vi "Serial Numbers.vi"(11 "Total Number of Units":i32=1 min=1 max=32 step=1) -> (2 "Serial Numbers":string[](array[string]))   [LabVIEW 2024]
panel:
  in  "Serial Number":string
  in  "Enter":bool
  out "Current Unit":i32
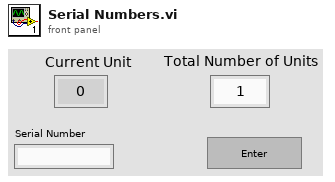
[diagram p1: front panel]
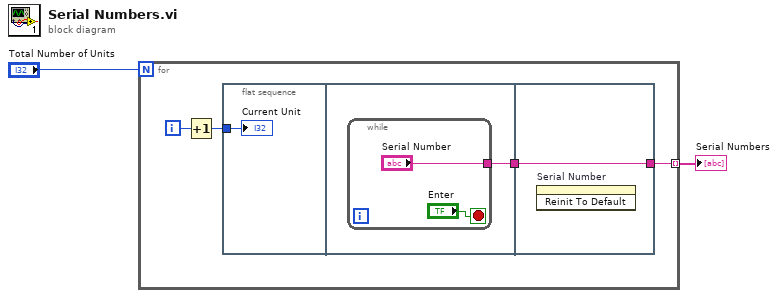
[diagram p0: block diagram]
diagram:
  n1 = for {
    N: "Total Number of Units" -> [_]
    tunnel: [w6] -> w1 mode=indexing
    i -> [w5]
    n2 = Increment(x=w5) -> (x+1=w4:i32)
    n3 = flat-sequence {
      tunnel: w4 -> [w7]
      tunnel: [w8] -> w3
      tunnel: [w11] -> w6
      tunnel: w3 -> [w11]
      frame #0 {
        "Current Unit" <- w7
      }
      frame #1 {
        n4 = while {
          tunnel: ["Serial Number"] -> w8
          stop <- "Enter" stop-if-true
        }
      }
      frame #2 {
        n5 = invoke on="Serial Number" class="Str" method="Reinit To Default"() -> ()  [unwired: 3 in, 3 out]
      }
    }
  }
  "Serial Numbers" <- w1
